vi "red_buoy_threshing_particle.vi"(8 "Image":T1, 9 "error in (no error)":errorcluster) -> (0 "error out":errorcluster, 3 "Image Out":T1(plugin-control))   [LabVIEW 2009]
uses:
  <vilib>/vision/Image Controls.llb/IMAQ Image.ctl
  <vilib>/vision/NI_Vision_Development_Module.lvlib
panel:
  out "min circularity":dbl[](array[numeric])
  out "circularities":dbl[](array[numeric])
  out "Particle Measurements (Pixels)":dbl[][](array[numeric]) format="%.2f"
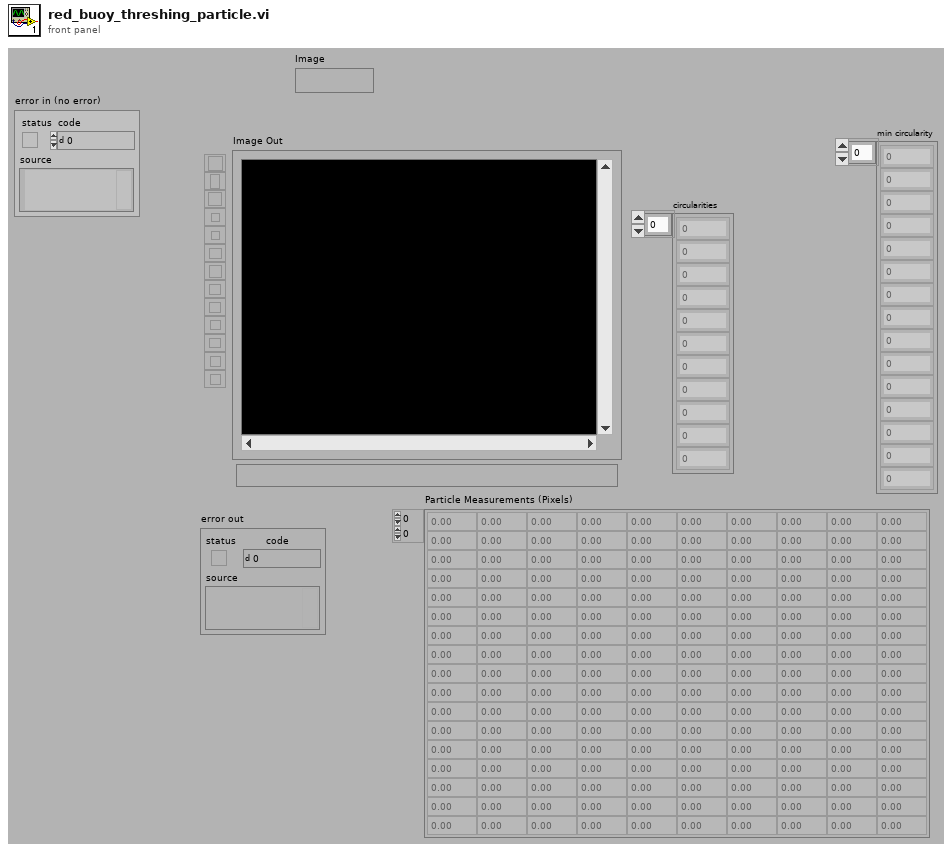
[diagram p1: front panel]
types:
  T1 = typedef "IMAQ Image.ctl" = refnum<image>
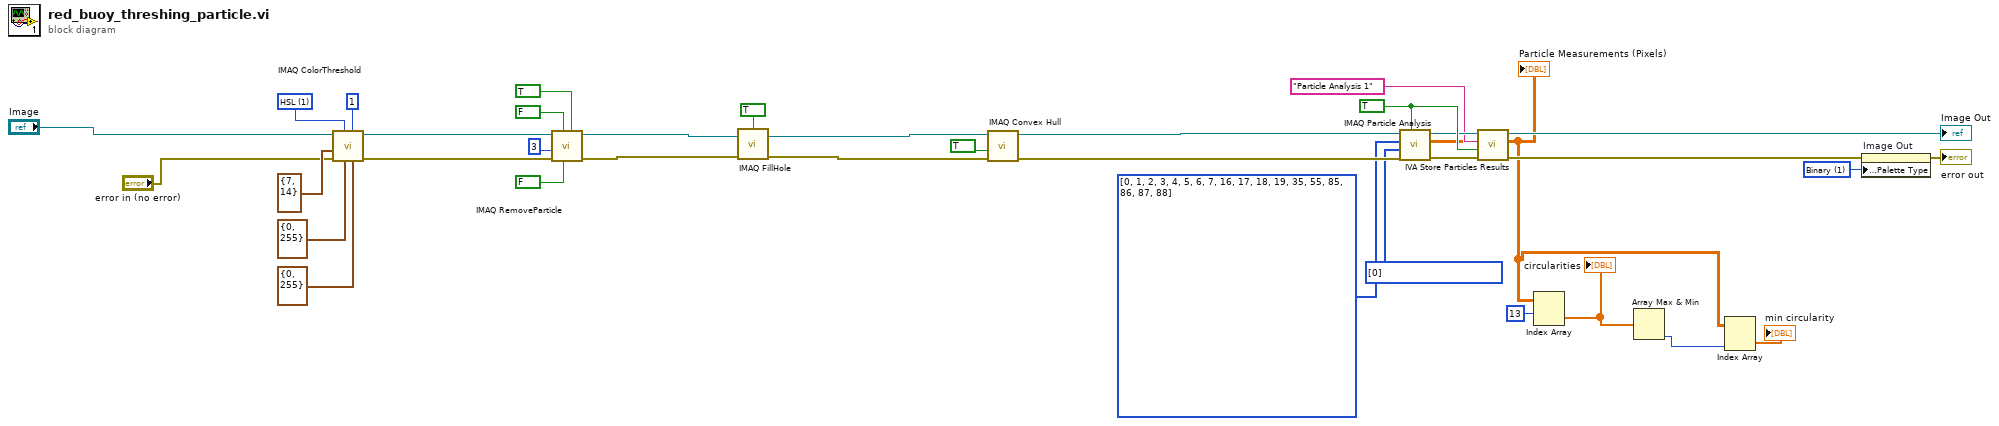
[diagram p0: block diagram]
diagram:
  w10 = u32 1 items=["Grayscale", "Binary", "Gradient", "Rainbow", "Temperature", "User Defined"] ("Palette")
  w18 = i32[] [0] items=["Center of Mass X", "Center of Mass Y", "First Pixel X", "First Pixel Y", "Bounding Rect Left", "Bounding Rect Top", "Bounding Rect Right", "Bounding Rect Bottom", "Max Feret Diameter Start X", "Max Feret Diameter Start Y", "Max Feret Diameter End X", "Max Feret Diameter End Y", "Max Horiz. Segment Length Left", "Max Horiz. Segment Length Right", "Max Horiz. Segment Length Row", "-", "Bounding Rect Width", "Bounding Rect Height", "Bounding Rect Diagonal", "Perimeter", "Convex Hull Perimeter", "Holes' Perimeter", "Max Feret Diameter", "Equivalent Ellipse Major Axis", "Equivalent Ellipse Minor Axis", "Equivalent Ellipse Minor Axis (Feret)", "Equivalent Rect Long Side", "Equivalent Rect Short Side", "Equivalent Rect Diagonal", "Equivalent Rect Short Side (Feret)", "Average Horiz. Segment Length", "Average Vert. Segment Length", "Hydraulic Radius", "Waddel Disk Diameter", "-", "Area", "Holes' Area", "Particle & Holes' Area", "Convex Hull Area", "Image Area", "-", "Number of Holes", "Number of Horiz. Segments", "Number of Vert. Segments", "-", "Orientation", "Max Feret Diameter Orientation", "-", "% Area/Image Area", "% Area/(Particle & Holes' Area)", "Ratio of Equivalent Ellipse Axes", "Ratio of Equivalent Rect Sides", "-", "Elongation Factor", "Compactness Factor", "Heywood Circularity Factor", "Type Factor", "-", "Sum X", "Sum Y", "Sum XX", "Sum XY", "Sum YY", "Sum XXX", "Sum XXY", "Sum XYY", "Sum YYY", "-", "Moment of Inertia XX", "Moment of Inertia XY", "Moment of Inertia YY", "Moment of Inertia XXX", "Moment of Inertia XXY", "Moment of Inertia XYY", "Moment of Inertia YYY", "Norm. Moment of Inertia XX", "Norm. Moment of Inertia XY", "Norm. Moment of Inertia YY", "Norm. Moment of Inertia XXX", "Norm. Moment of Inertia XXY", "Norm. Moment of Inertia XYY", "Norm. Moment of Inertia YYY", "Hu Moment 1", "Hu Moment 2", "Hu Moment 3", "Hu Moment 4", "Hu Moment 5", "Hu Moment 6", "Hu Moment 7"] ("Real-World Measurements")
  w6 = i32[] [0, 1, 2, 3, 4, 5, 6, 7, 16, 17, 18, 19, 35, 55, 85, 86, 87, 88] items=["Center of Mass X", "Center of Mass Y", "First Pixel X", "First Pixel Y", "Bounding Rect Left", "Bounding Rect Top", "Bounding Rect Right", "Bounding Rect Bottom", "Max Feret Diameter Start X", "Max Feret Diameter Start Y", "Max Feret Diameter End X", "Max Feret Diameter End Y", "Max Horiz. Segment Length Left", "Max Horiz. Segment Length Right", "Max Horiz. Segment Length Row", "-", "Bounding Rect Width", "Bounding Rect Height", "Bounding Rect Diagonal", "Perimeter", "Convex Hull Perimeter", "Holes' Perimeter", "Max Feret Diameter", "Equivalent Ellipse Major Axis", "Equivalent Ellipse Minor Axis", "Equivalent Ellipse Minor Axis (Feret)", "Equivalent Rect Long Side", "Equivalent Rect Short Side", "Equivalent Rect Diagonal", "Equivalent Rect Short Side (Feret)", "Average Horiz. Segment Length", "Average Vert. Segment Length", "Hydraulic Radius", "Waddel Disk Diameter", "-", "Area", "Holes' Area", "Particle & Holes' Area", "Convex Hull Area", "Image Area", "-", "Number of Holes", "Number of Horiz. Segments", "Number of Vert. Segments", "-", "Orientation", "Max Feret Diameter Orientation", "-", "% Area/Image Area", "% Area/(Particle & Holes' Area)", "Ratio of Equivalent Ellipse Axes", "Ratio of Equivalent Rect Sides", "-", "Elongation Factor", "Compactness Factor", "Heywood Circularity Factor", "Type Factor", "-", "Sum X", "Sum Y", "Sum XX", "Sum XY", "Sum YY", "Sum XXX", "Sum XXY", "Sum XYY", "Sum YYY", "-", "Moment of Inertia XX", "Moment of Inertia XY", "Moment of Inertia YY", "Moment of Inertia XXX", "Moment of Inertia XXY", "Moment of Inertia XYY", "Moment of Inertia YYY", "Norm. Moment of Inertia XX", "Norm. Moment of Inertia XY", "Norm. Moment of Inertia YY", "Norm. Moment of Inertia XXX", "Norm. Moment of Inertia XXY", "Norm. Moment of Inertia XYY", "Norm. Moment of Inertia YYY", "Hu Moment 1", "Hu Moment 2", "Hu Moment 3", "Hu Moment 4", "Hu Moment 5", "Hu Moment 6", "Hu Moment 7"] ("Pixel Measurements")
  w16 = TRUE ("Connectivity 4/8 (8)")
  w35 = u16 1 items=["RGB", "HSL", "HSV", "HSI"] ("Color Mode")
  n1 = call "IMAQ ColorThreshold"("Blue or Luma or Val or Inten Range"=cluster{"Lower value":i32, "Upper value":i32} {"Lower value"=0, "Upper value"=255}, "Replace Value"=1, "Green or Sat Range"=cluster{"Lower value":i32, "Upper value":i32} {"Lower value"=0, "Upper value"=255}, "Color Mode"=w35, "error in (no error)"="error in (no error)", "Red or Hue Range"=cluster{"Lower value":i32, "Upper value":i32} {"Lower value"=7, "Upper value"=14}, "Image Src"="Image") -> ("error out"=w31:errorcluster, "Image Dst Out"=w26:T1)  [unwired: 1 in, 2 out]
  n2 = call "IMAQ RemoveParticle"("Connectivity 4/8 (8)"=TRUE, "Low Pass/High Pass (Low)"=FALSE, "Square/Hexa (Square)"=FALSE, "error in (no error)"=w31, "Number of Erosion"=3, "Image Src"=w26) -> ("error out"=w25:errorcluster, "Image Dst Out"=w23:T1)  [unwired: 1 in, 3 out]
  n3 = call "IMAQ FillHole"("error in (no error)"=w25, "Image Src"=w23, "Connectivity 4/8 (8)"=TRUE) -> ("error out"=w22:errorcluster, "Image Dst Out"=w21:T1)  [unwired: 1 in, 2 out]
  n4 = call "IMAQ Convex Hull"("error in (no error)"=w22, "Connectivity 4/8 (8)"=TRUE, "Image Src"=w21) -> ("error out"=w19:errorcluster, "Image Dst Out"=w17:T1)  [unwired: 1 in, 6 out]
  n5 = call "IMAQ Particle Analysis"("Connectivity 4/8 (8)"=w16, "error in (no error)"=w19, "Real-World Measurements"=w18, "Pixel Measurements"=w6, "Image"=w17) -> ("error out"=w13:errorcluster, "Particle Measurements (Pixels)"=w3:dbl[][], "Image Out (duplicate)"=w15:T1)  [unwired: 4 out]
  "Particle Measurements (Pixels)" <- w3
  n6 = call <vilib>:"IVA Store Particles Results.vi"("error in (no error)"=w13, "Connectivity 4/8 (8)"=w16, "Step Name"="Particle Analysis 1", "Image in"=w15) -> ("error out"=w12:errorcluster, "Image dup"=→"Image Out":T1)  [unwired: 6 out]
  n7 = Index Array(array=w3, index (row)=13) -> (element=w4:dbl[])  [unwired: 1 in]
  "circularities" <- w4
  n8 = Array Max & Min(array=w4) -> (min index (indices)=w2:i32)  [unwired: 3 out]
  n9 = Index Array(array=w3, index (col)=w2) -> (element=→"min circularity":dbl[])  [unwired: 1 in]
  n10 = property on="Image Out" class="ImageControl"(error in=w12, "Palette:Palette Type"=w10) -> (error out=→"error out":errorcluster)  [unwired: 1 in, 1 out]
